vi "SubModule RENAME ME.vi"(8 "Error in":errorcluster, 11 "External Event":refnum<user-event>) -> (0 "Error out":errorcluster)   [LabVIEW 2018, in "QMH Template.lvlib"]
uses:
  QMH Template.lvlib
  Event Messaging/Type Defs/Event Message--cluster.ctl
  Type Defs/Data--cluster.ctl
  QMH/QMH CORE.lvlib
  Queue Messaging/Queue Messaging.lvlib
  Event Messaging/Event Messaging.lvlib
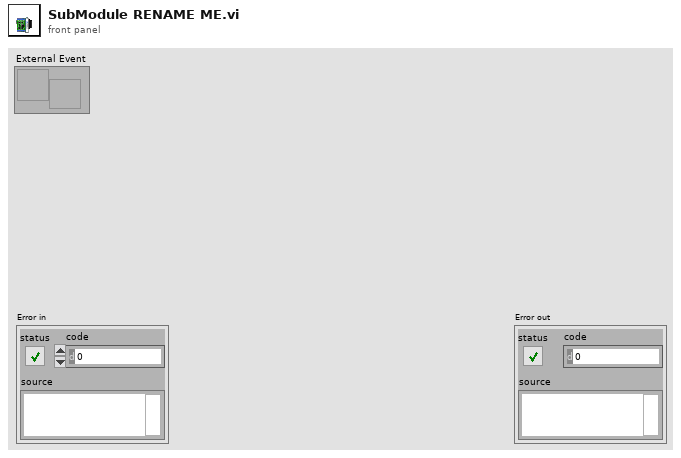
[diagram p1: front panel]
types:
  T1 = typedef "QMH Template.lvlib/Data--cluster.ctl" = cluster{"String":string}
  T2 = typedef "QMH CORE.lvlib/EventsAndQueues--cluster.ctl" = cluster{"Internal Queue":refnum<queue>, "Internal Event":refnum<user-event>, "External Event":refnum<user-event>}
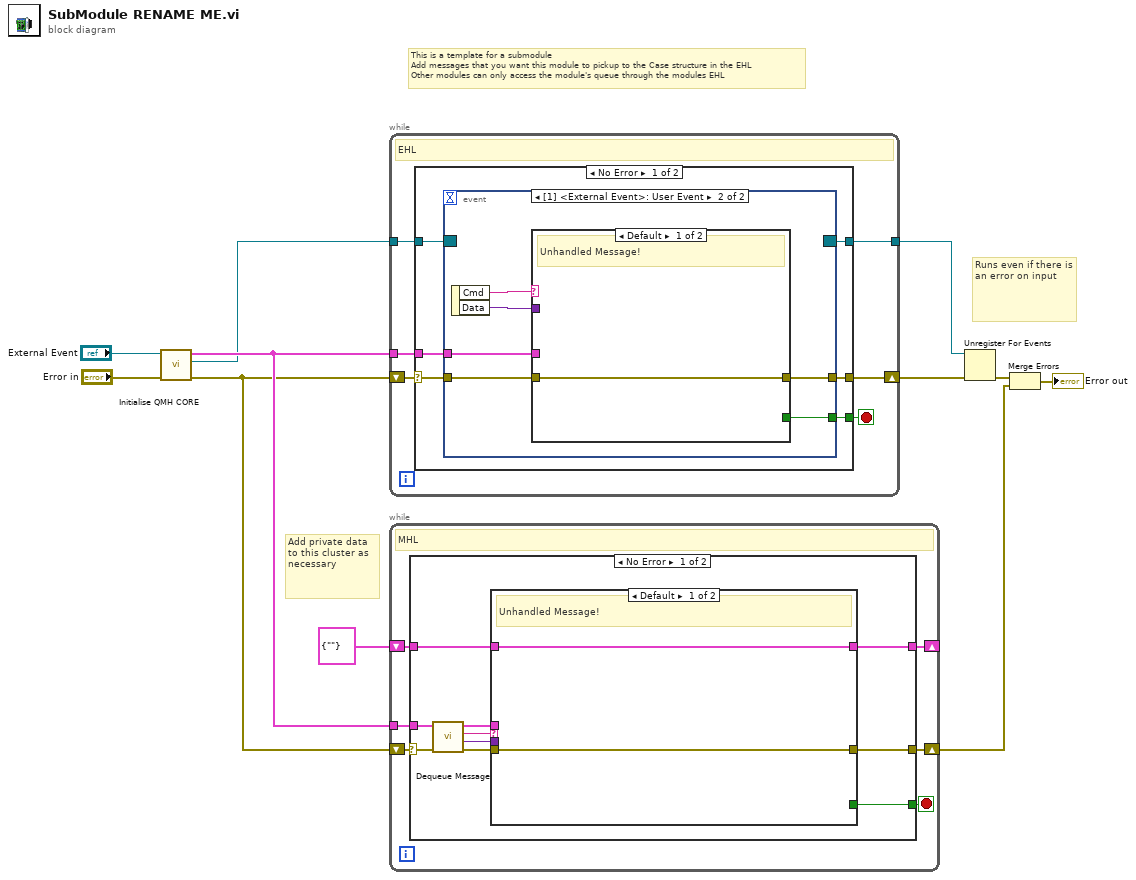
[diagram p0: block diagram]
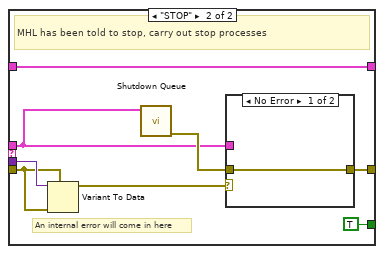
[diagram p2: hidden frame]
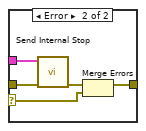
[diagram p3: hidden frame]
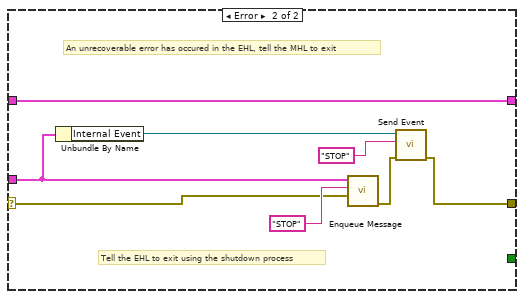
[diagram p4: hidden frame]
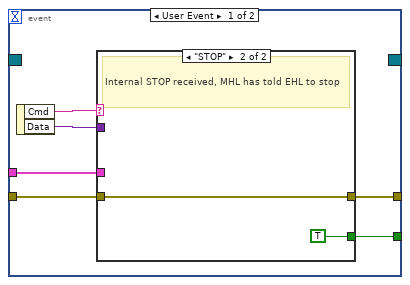
[diagram p5: hidden frame]
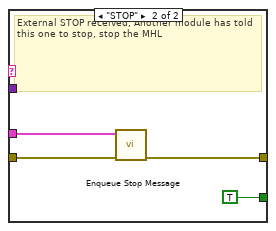
[diagram p7: hidden frame]
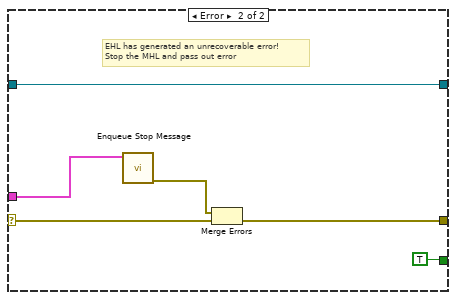
[diagram p8: hidden frame]
diagram:
  # "Add private data to this cluster as necessary"
  # "This is a template for a submodule\nAdd messages that you want this module to pickup to the Case structure in the EHL\nOther modules can only access the module's queue through the modules EHL"
  # "Runs even if there is an error on input"
  n1 = call "Initialise QMH CORE.vi"("Error in"="Error in", "External Event"="External Event") -> ("Error out"=w10:errorcluster, "Event Registration Refnum"=w9:refnum<event-registration>, "Queue Data"=w11:T2)  [unwired: 7 in]
  n2 = while {
    shift-right: [w15] -> w8
    shift-left: w10 -> [w17]
    tunnel: w11 -> [w16]
    tunnel: w9 -> [w13]
    tunnel: [w12] -> w7
    stop <- w14 stop-if-true
    # "EHL"
    n3 = case shown="No Error" w17 {
      selector: w17 -> [w23 w48]
      tunnel: w16 -> [w22 w49]
      tunnel: [w21 w45] -> w15
      tunnel: [w20 TRUE] -> w14
      tunnel: w13 -> [w19 w46]
      tunnel: [w18 w46] -> w12
      frame No Error {
        n4 = event shown="[1] <External Event>: User Event" {
          selector: w19 -> [_ _]
          dyn-events: [_ _] -> w18
          timeout: _ -> [_ _]
          tunnel: w23 -> [w29 w36]
          tunnel: w22 -> [w25 w33]
          tunnel: [w28 w35] -> w21
          tunnel: [w24 w34] -> w20
          event User Event {
            n5 = event-data() -> ("Cmd"=w27:string, "Data"=w26:variant)  [unwired: 1 in]
            n6 = case shown="\"STOP\"" w27 {
              tunnel: w29 -> [w30 w31]
              tunnel: [w30 w31] -> w28
              tunnel: w26 -> [_ _]
              tunnel: w25 -> [_ _]
              tunnel: [_ TRUE] -> w24
              frame Default {
                # "Unhandled Message!"
              }
              frame "STOP" {
                # "Internal STOP received, MHL has told EHL to stop"
              }
            }
          }
          event User Event {
            n7 = event-data() -> ("Cmd"=w38:string, "Data"=w37:variant)  [unwired: 1 in]
            n8 = case shown="Default" w38 {
              tunnel: w36 -> [w39 w42]
              tunnel: [w39 w41] -> w35
              tunnel: [_ TRUE] -> w34
              tunnel: w37 -> [_ _]
              tunnel: w33 -> [_ w40]
              frame Default {
                # "Unhandled Message!"
              }
              frame "STOP" {
                # "External STOP received, Another module has told this one to stop, stop the MHL"
                n9 = call "Enqueue Stop Message.vi"("Error in"=w42, "Queue Data"=w40) -> ("Error out"=w41:errorcluster)  [unwired: 9 in]
              }
            }
          }
        }
      }
      frame Error {
        # "EHL has generated an unrecoverable error!\nStop the MHL and pass out error"
        n10 = call "Enqueue Stop Message.vi"("Queue Data"=w49) -> ("Error out"=w44:errorcluster)  [unwired: 10 in]
        n11 = Merge Errors(w44, w48) -> (w45:errorcluster)
      }
    }
  }
  n12 = while {
    shift-right: [w53] -> w3
    shift-left: w10 -> [w55]
    tunnel: w11 -> [w54]
    shift-right: [w51] -> _
    shift-left: T1 {"String"=""} -> [w50]
    stop <- w52 stop-if-true
    # "MHL"
    n13 = case shown="No Error" w55 {
      selector: w55 -> [w65 w85]
      tunnel: w54 -> [w64 w87]
      tunnel: [w60 w83] -> w53
      tunnel: [w59 _] -> w52
      tunnel: [w57 w82] -> w51
      tunnel: w50 -> [w56 w82]
      frame No Error {
        n14 = call "Dequeue Message.vi"("Error in"=w65, "Queue Data in"=w64) -> ("Error out"=w62:errorcluster, "Data"=w61:variant, "Cmd"=w63:string, "Queue Data out"=w58:T2)  [unwired: 6 in]
        n15 = case shown="Default" w63 {
          tunnel: w62 -> [w67 w73]
          tunnel: w61 -> [_ w74]
          tunnel: [w67 w70] -> w60
          tunnel: [_ TRUE] -> w59
          tunnel: w58 -> [_ w69]
          tunnel: [w66 w68] -> w57
          tunnel: w56 -> [w66 w68]
          frame Default {
            # "Unhandled Message!"
          }
          frame "STOP" {
            # "An internal error will come in here"
            # "MHL has been told to stop, carry out stop processes"
            n16 = Variant To Data(error in=w73, type=w73, Variant=w74) -> (data=w72:errorcluster)  [unwired: 1 out]
            n17 = call "Shutdown Queue.vi"("Queue Data"=w69) -> ("Error out"=w71:errorcluster)  [unwired: 10 in]
            n18 = case shown="No Error" w72 {
              selector: w72 -> [_ w77]
              tunnel: w71 -> [w76 w81]
              tunnel: [w76 w79] -> w70
              tunnel: w69 -> [_ w80]
              frame No Error {
              }
              frame Error {
                n19 = call "Send Internal Stop.vi"("Error in"=w81, "Queue Data"=w80) -> ("Error out"=w78:errorcluster)  [unwired: 9 in]
                n20 = Merge Errors(w78, w77) -> (w79:errorcluster)
              }
            }
          }
        }
      }
      frame Error {
        # "Tell the EHL to exit using the shutdown process"
        # "An unrecoverable error has occured in the EHL, tell the MHL to exit"
        n21 = Unbundle By Name(w87) -> ("Internal Event"=w89:refnum<user-event>)
        n22 = call "Enqueue Message.vi"("Data"=w85, "Cmd"="STOP", "Queue Data"=w87) -> ("Error out"=w84:errorcluster)  [unwired: 8 in]
        n23 = call "Send Event.vi"("Error in"=w84, "Cmd"="STOP", "Event Ref"=w89) -> ("Error out"=w83:errorcluster)  [unwired: 7 in, 1 out]
      }
    }
  }
  n24 = Unregister For Events(event registration refnum=w7, error in=w8) -> (error out=w5:errorcluster)
  n25 = Merge Errors(w5, w3) -> (→"Error out":errorcluster)
